vi "Saturation transfer-v2.vi"() -> ()   [LabVIEW 2016]
uses:
  <vilib>/Analysis/6fits.llb/Curve Fitting Criteria.ctl
  <vilib>/Utility/file.llb/Write To Spreadsheet File (string).vi
  <vilib>/Utility/file.llb/Write To Spreadsheet File (DBL).vi
  Driver/New driver/Agilent 415X Series.lvlib
  <vilib>/Analysis/NI_AALPro.lvlib
panel:
  out "power":dbl
  in  "short int. time":dbl(knob)=0.00064 scale=8e-05..0.00056
  in  "integration time":i32(slide) scale=0.0..2.0
  out "error out":errorcluster
  out "error":i32
  in  "parameter bounds":T1={"amp min"=-inf, "amp max"=inf, "power min"=-inf, "power max"=inf, "offset min"=0.0, "offset max"=0.0}
  in  "Dielectric thickness (nm)":dbl
  in  "Dielectric constant":dbl
  in  "Channel length (mm)":dbl
  in  "Channel width (mm)":dbl
  out "Graph  3":cluster{"Output data":dbl[], dbl[]}(graph) caption="Mobility Calculation"
  out "Graph  2":cluster{"Output data":dbl[], dbl[]}[](graph) caption="SMU 2 (ID) & SMU 3 (IG)"
  in  "LINEAR STEP":dbl
  in  "STOP":dbl
  in  "START":dbl
  in  "RATIO":dbl
  in  "OFFSET":dbl
  in  "FILE PATH":path
  out "SPA VISA resource name  End":refnum<visa-resource-name>
  in  "SPA VISA resource name Start":refnum<visa-resource-name>="GPIB0::14::INSTR"
  in  "error in (no error)":errorcluster
  # "SMU 3: Gate \nSMU3 = SMU2*RATIO\n             +OFFSET"
  # "SMU 1: Source"
  # "Common"
  # "SMU 2: Drain"
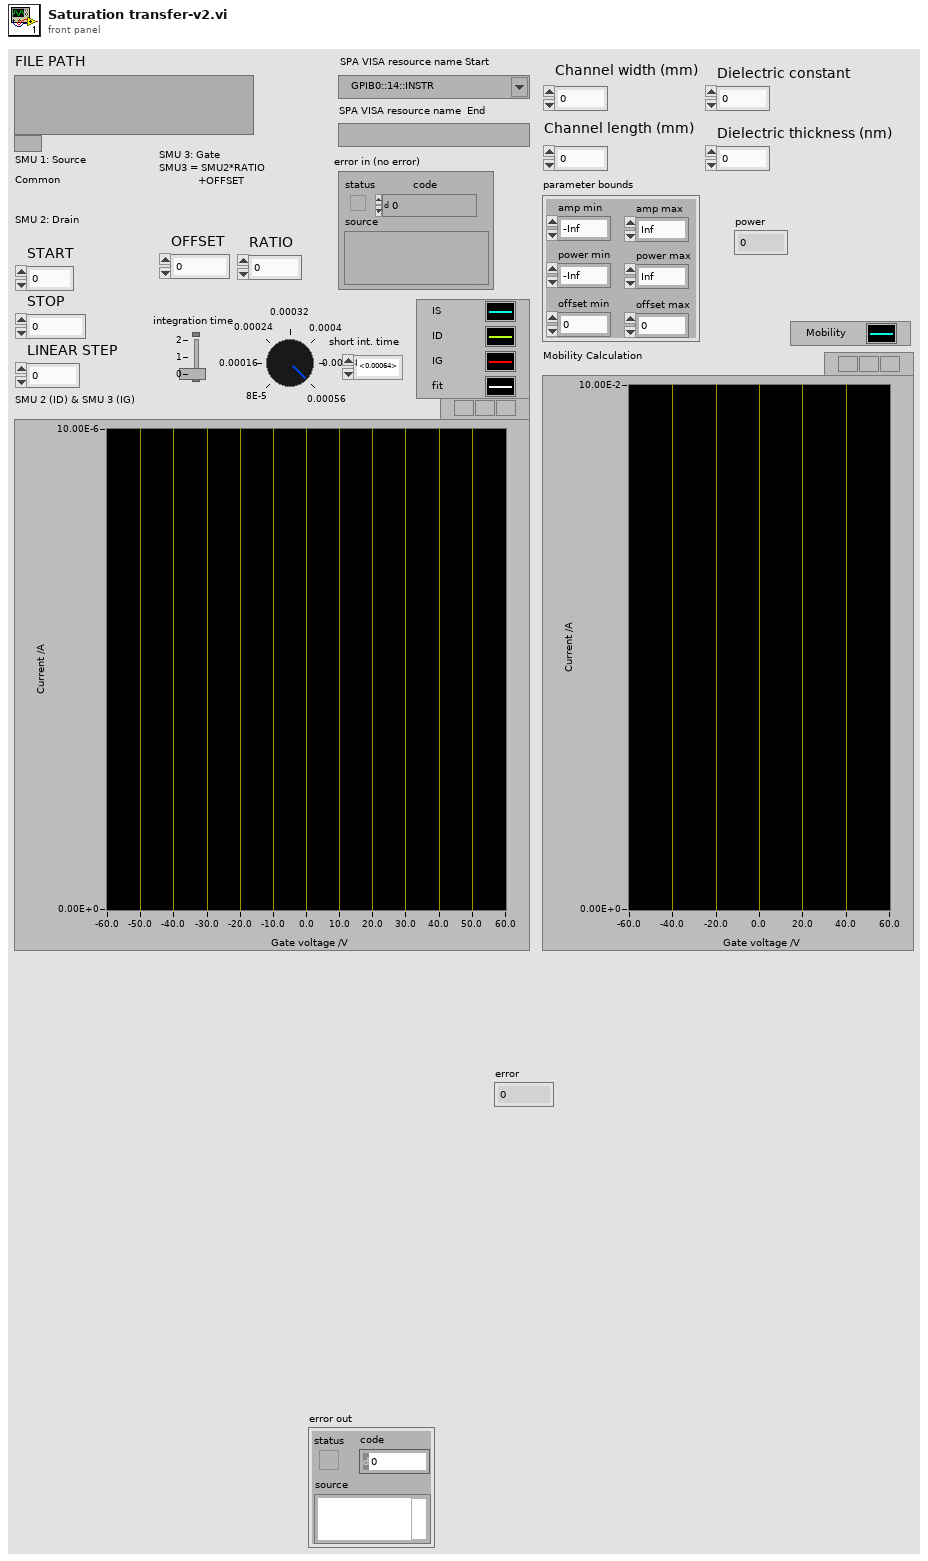
[diagram p1: front panel]
types:
  T1 = cluster{"amp min":dbl, "amp max":dbl, "power min":dbl, "power max":dbl, "offset min":dbl, "offset max":dbl}
  T2 = typedef "NI_AALPro.lvlib/Curve Fitting Criteria.ctl" = u16
  T3 = cluster{"Output data":dbl[], "Best Power Fit":dbl[]}[]
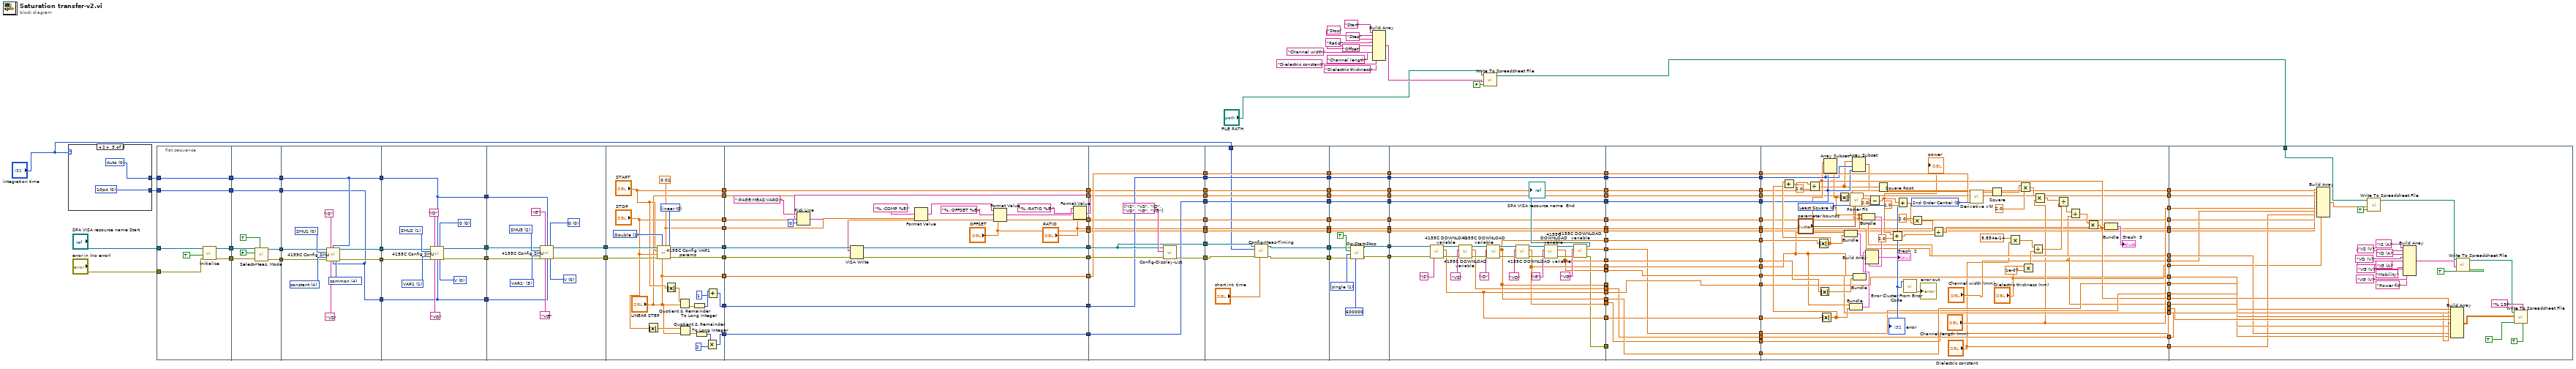
[diagram p0: block diagram]
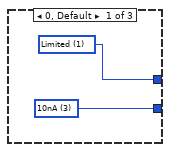
[diagram p2: hidden frame]
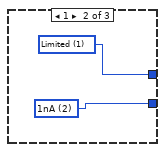
[diagram p3: hidden frame]
diagram:
  n1 = case shown="2" "integration time" {
    tunnel: [w143 w145 w147] -> w8
    tunnel: [w142 w144 w146] -> w4
    frame 0, Default {
      w142 = u8 3 items=["10pA  ", "100pA  ", "1nA  ", "10nA", "100nA", "1uA", "10uA", "100uA", "1mA", "10mA", "100mA", "1A"] ("Range")
      w143 = u16 1 items=["Auto", "Limited", "Fixed"] ("Range mode")
    }
    frame 1 {
      w144 = u8 2 items=["10pA  ", "100pA  ", "1nA  ", "10nA", "100nA", "1uA", "10uA", "100uA", "1mA", "10mA", "100mA", "1A"] ("Range")
      w145 = u16 1 items=["Auto", "Limited", "Fixed"] ("Range mode")
    }
    frame 2 {
      w146 = u8 0 items=["10pA  ", "100pA  ", "1nA  ", "10nA", "100nA", "1uA", "10uA", "100uA", "1mA", "10mA", "100mA", "1A"] ("Range")
      w147 = u16 0 items=["Auto", "Limited", "Fixed"] ("Range mode")
    }
  }
  n2 = flat-sequence {
    tunnel: "error in (no error)" -> [w153]
    tunnel: "SPA VISA resource name Start" -> [w152]
    tunnel: [w151] -> w141
    tunnel: [w150] -> w140
    tunnel: w8 -> [w149]
    tunnel: [w149] -> w7
    tunnel: w4 -> [w148]
    tunnel: [w148] -> w2
    tunnel: w141 -> [w162]
    tunnel: w140 -> [w161]
    tunnel: [w158] -> w139
    tunnel: [w157] -> w138
    tunnel: w7 -> [w156]
    tunnel: [w156] -> w6
    tunnel: [w155] -> w3
    tunnel: w2 -> [w155]
    tunnel: w139 -> [w168]
    tunnel: w138 -> [w166]
    tunnel: [w167] -> w133
    tunnel: [w165] -> w132
    tunnel: [w163] -> w114
    tunnel: w6 -> [w164]
    tunnel: [w164] -> w5
    tunnel: w3 -> [w163]
    tunnel: [w185] -> w137
    tunnel: [w184] -> w136
    tunnel: w133 -> [w178]
    tunnel: w132 -> [w177]
    tunnel: [w174] -> w118
    tunnel: w114 -> [w175]
    tunnel: [w175] -> w113
    tunnel: w5 -> [w174]
    tunnel: w136 -> [w191]
    tunnel: w137 -> [w192]
    tunnel: [w189] -> w131
    tunnel: [w188] -> w130
    tunnel: w118 -> [w187]
    tunnel: w113 -> [w186]
    tunnel: w131 -> [w217]
    tunnel: w130 -> [w216]
    tunnel: [w213] -> w117
    tunnel: [w212] -> w116
    tunnel: [w211] -> w115
    tunnel: ["LINEAR STEP"] -> w95
    tunnel: [w201] -> w88
    tunnel: [w206] -> w81
    tunnel: ["START"] -> w45
    tunnel: ["STOP"] -> w37
    tunnel: ["LINEAR STEP"] -> w29
    tunnel: w117 -> [w237]
    tunnel: [w236] -> w108
    tunnel: w116 -> [w239]
    tunnel: [w238] -> w107
    tunnel: w115 -> [w233]
    tunnel: [w225] -> w96
    tunnel: w95 -> [w225]
    tunnel: [w224] -> w89
    tunnel: w88 -> [w224]
    tunnel: [w223] -> w82
    tunnel: w81 -> [w223]
    tunnel: [w222] -> w46
    tunnel: w45 -> [w222]
    tunnel: [w221] -> w38
    tunnel: w37 -> [w221]
    tunnel: [w220] -> w30
    tunnel: w29 -> [w220]
    tunnel: ["RATIO"] -> w22
    tunnel: ["OFFSET"] -> w15
    tunnel: w108 -> [w248]
    tunnel: w107 -> [w249]
    tunnel: [w250] -> w106
    tunnel: [w248] -> w105
    tunnel: [w247] -> w97
    tunnel: w96 -> [w247]
    tunnel: [w246] -> w90
    tunnel: w89 -> [w246]
    tunnel: [w245] -> w83
    tunnel: w82 -> [w245]
    tunnel: [w244] -> w47
    tunnel: w46 -> [w244]
    tunnel: [w243] -> w39
    tunnel: w38 -> [w243]
    tunnel: [w242] -> w31
    tunnel: w30 -> [w242]
    tunnel: [w241] -> w23
    tunnel: w22 -> [w241]
    tunnel: [w240] -> w16
    tunnel: w15 -> [w240]
    tunnel: w106 -> [w255]
    tunnel: w105 -> [w257]
    tunnel: [w265] -> w98
    tunnel: w97 -> [w265]
    tunnel: [w264] -> w91
    tunnel: w90 -> [w264]
    tunnel: [w263] -> w84
    tunnel: w83 -> [w263]
    tunnel: [w262] -> w48
    tunnel: w47 -> [w262]
    tunnel: [w261] -> w40
    tunnel: w39 -> [w261]
    tunnel: [w260] -> w32
    tunnel: w31 -> [w260]
    tunnel: [w259] -> w24
    tunnel: w23 -> [w259]
    tunnel: [w258] -> w17
    tunnel: w16 -> [w258]
    tunnel: [w256] -> w10
    tunnel: [w254] -> w9
    tunnel: "integration time" -> [w253]
    tunnel: [w277] -> w110
    tunnel: [w276] -> w109
    tunnel: [w275] -> w99
    tunnel: w98 -> [w275]
    tunnel: [w274] -> w92
    tunnel: w91 -> [w274]
    tunnel: [w273] -> w85
    tunnel: w84 -> [w273]
    tunnel: [w272] -> w49
    tunnel: w48 -> [w272]
    tunnel: [w271] -> w41
    tunnel: w40 -> [w271]
    tunnel: [w270] -> w33
    tunnel: w32 -> [w270]
    tunnel: [w269] -> w25
    tunnel: w24 -> [w269]
    tunnel: [w268] -> w18
    tunnel: w17 -> [w268]
    tunnel: w10 -> [w267]
    tunnel: w9 -> [w266]
    tunnel: [w289] -> w129
    tunnel: [w296] -> w128
    tunnel: [w293] -> w127
    tunnel: [w295] -> w126
    tunnel: [w294] -> w125
    tunnel: [w298] -> w124
    tunnel: [w293] -> w123
    tunnel: [w295] -> w121
    tunnel: [w294] -> w119
    tunnel: [w293] -> w112
    tunnel: w110 -> [w292]
    tunnel: w109 -> [w291]
    tunnel: [w290] -> w104
    tunnel: [w289] -> w102
    tunnel: [w288] -> w100
    tunnel: w99 -> [w288]
    tunnel: [w287] -> w93
    tunnel: w92 -> [w287]
    tunnel: [w286] -> w86
    tunnel: w85 -> [w286]
    tunnel: [w285] -> w50
    tunnel: w49 -> [w285]
    tunnel: [w284] -> w42
    tunnel: w41 -> [w284]
    tunnel: [w283] -> w34
    tunnel: w33 -> [w283]
    tunnel: [w282] -> w26
    tunnel: w25 -> [w282]
    tunnel: [w281] -> w19
    tunnel: w18 -> [w281]
    tunnel: w129 -> [w325]
    tunnel: w128 -> [w324]
    tunnel: w127 -> [w323]
    tunnel: w126 -> [w322]
    tunnel: w125 -> [w321]
    tunnel: w124 -> [w320]
    tunnel: w123 -> [_]
    tunnel: [w332] -> w122
    tunnel: w121 -> [w332]
    tunnel: [w331] -> w120
    tunnel: w119 -> [w331]
    tunnel: w112 -> [w330]
    tunnel: [w330] -> w111
    tunnel: w104 -> [_]
    tunnel: [w329] -> w103
    tunnel: w102 -> [w329]
    tunnel: [w328] -> w101
    tunnel: w100 -> [w328]
    tunnel: [w327] -> w94
    tunnel: w93 -> [w327]
    tunnel: [w326] -> w87
    tunnel: w86 -> [w326]
    tunnel: [w325] -> w79
    tunnel: [w324] -> w77
    tunnel: [w323] -> w75
    tunnel: [w322] -> w73
    tunnel: [w321] -> w71
    tunnel: [w320] -> w69
    tunnel: [w319] -> w51
    tunnel: w50 -> [w319]
    tunnel: [w318] -> w43
    tunnel: w42 -> [w318]
    tunnel: [w317] -> w35
    tunnel: w34 -> [w317]
    tunnel: [w316] -> w27
    tunnel: w26 -> [w316]
    tunnel: [w315] -> w20
    tunnel: w19 -> [w315]
    tunnel: w122 -> [w345]
    tunnel: w120 -> [w398]
    tunnel: w111 -> [w399]
    tunnel: w103 -> [w395]
    tunnel: w101 -> [w383]
    tunnel: w94 -> [w359]
    tunnel: w87 -> [w358]
    tunnel: [w354] -> w80
    tunnel: w79 -> [w354]
    tunnel: [w353] -> w78
    tunnel: w77 -> [w353]
    tunnel: [w352] -> w76
    tunnel: w75 -> [w352]
    tunnel: [w351] -> w74
    tunnel: w73 -> [w351]
    tunnel: [w350] -> w72
    tunnel: w71 -> [w350]
    tunnel: [w349] -> w70
    tunnel: w69 -> [w349]
    tunnel: [w348] -> w68
    tunnel: [w347] -> w67
    tunnel: [w346] -> w66
    tunnel: [w344] -> w52
    tunnel: w51 -> [w344]
    tunnel: [w343] -> w44
    tunnel: w43 -> [w343]
    tunnel: [w342] -> w36
    tunnel: w35 -> [w342]
    tunnel: [w341] -> w28
    tunnel: w27 -> [w341]
    tunnel: [w340] -> w21
    tunnel: w20 -> [w340]
    tunnel: ["Channel width (mm)"] -> w14
    tunnel: ["Channel length (mm)"] -> w13
    tunnel: ["Dielectric constant"] -> w12
    tunnel: ["Dielectric thickness (nm)"] -> w11
    tunnel: w80 -> [w433]
    tunnel: w78 -> [w432]
    tunnel: w76 -> [w431]
    tunnel: w74 -> [w430]
    tunnel: w72 -> [w429]
    tunnel: w70 -> [w428]
    tunnel: w68 -> [w427]
    tunnel: w67 -> [w426]
    tunnel: w66 -> [w425]
    tunnel: w53 -> [w402]
    tunnel: w52 -> [w412]
    tunnel: w44 -> [w411]
    tunnel: w36 -> [w410]
    tunnel: w28 -> [w409]
    tunnel: w21 -> [w408]
    tunnel: w14 -> [w407]
    tunnel: w13 -> [w406]
    tunnel: w12 -> [w405]
    tunnel: w11 -> [w404]
    frame #0 {
      n3 = call "Initialize.vi"("error in (no error)"=w153, "reset"=TRUE, "VISA resource name"=w152) -> ("error out"=w150:errorcluster, "VISA resource name out"=w151:refnum<visa-resource-name>)  [unwired: 2 in, 5 out]
    }
    frame #1 {
      n4 = call "Select-Meas. Mode.vi"("clear all channels"=TRUE, "error in (no error)"=w161, "measurement mode"=FALSE, "VISA resource name"=w162) -> ("error out"=w157:errorcluster, "VISA resource name out"=w158:refnum<visa-resource-name>)  [unwired: 1 in, 5 out]
    }
    frame #2 {
      w169 = u32 0 items=["SMU1  ", "SMU2  ", "SMU3  ", "SMU4  ", "SMU5  ", "SMU6  "] ("unit to configure")
      w170 = u32 4 items=["disabled  ", "VAR1  ", "VAR2  ", "VAR1'  ", "constant  "] ("function")
      w171 = u32 4 items=["V  ", "I  ", "V pulse  ", "I pulse  ", "  common  "] ("mode")
      n5 = call "4155C Config SMU.vi"("VISA session"=w168, "I name (max 6 chars)"="IS", "Range mode"=w164, "unit to configure"=w169, "function"=w170, "error in (no error)"=w166, "V name (max 6 chars)"="VS", "Range"=w163, "mode"=w171) -> ("dup VISA resource name"=w167:refnum<visa-resource-name>, "error out"=w165:errorcluster)  [unwired: 5 in]
    }
    frame #3 {
      w176 = u32 0 items=["0  ", "10K Ohms  ", "100K Ohms  ", "1M Ohms  "] ("series resistance *")
      w179 = u32 1 items=["SMU1  ", "SMU2  ", "SMU3  ", "SMU4  ", "SMU5  ", "SMU6  "] ("unit to configure")
      w180 = u32 1 items=["disabled  ", "VAR1  ", "VAR2  ", "VAR1'  ", "constant  "] ("function")
      w181 = u32 0 items=["V  ", "I  ", "V pulse  ", "I pulse  ", "  common  "] ("mode")
      n6 = call "4155C Config SMU.vi"("VISA session"=w178, "I name (max 6 chars)"="ID", "Range mode"=w174, "series resistance *"=w176, "unit to configure"=w179, "function"=w180, "error in (no error)"=w177, "V name (max 6 chars)"="VD", "Range"=w175, "mode"=w181) -> ("dup VISA resource name"=w185:refnum<visa-resource-name>, "error out"=w184:errorcluster)  [unwired: 4 in]
    }
    frame #4 {
      w190 = u32 0 items=["0  ", "10K Ohms  ", "100K Ohms  ", "1M Ohms  "] ("series resistance *")
      w193 = u32 2 items=["SMU1  ", "SMU2  ", "SMU3  ", "SMU4  ", "SMU5  ", "SMU6  "] ("unit to configure")
      w194 = u32 3 items=["disabled  ", "VAR1  ", "VAR2  ", "VAR1'  ", "constant  "] ("function")
      w195 = u32 0 items=["V  ", "I  ", "V pulse  ", "I pulse  ", "  common  "] ("mode")
      n7 = call "4155C Config SMU.vi"("VISA session"=w192, "I name (max 6 chars)"="IG", "Range mode"=w187, "series resistance *"=w190, "unit to configure"=w193, "function"=w194, "error in (no error)"=w191, "V name (max 6 chars)"="VG", "Range"=w186, "mode"=w195) -> ("dup VISA resource name"=w189:refnum<visa-resource-name>, "error out"=w188:errorcluster)  [unwired: 4 in]
    }
    frame #5 {
      w211 = 0.01 ("compliance")
      w214 = u16 1 items=["Single", "Double"] ("sweep mode")
      w215 = u16 0 items=["linear", "log 10", "log 25", "log 50"] ("sweep spacing (linear: 0)")
      n8 = Absolute Value(x="STOP") -> (abs(x)=w204:dbl)
      n9 = call "4155C Config VAR1 params.vi"("sweep spacing (linear: 0)"=w215, "compliance"=w211, "step (linear only)"="LINEAR STEP", "sweep mode"=w214, "error in (no error)"=w216, "stop"="STOP", "start"="START", "VISA session"=w217) -> ("error out"=w212:errorcluster, "dup VISA resource name"=w213:refnum<visa-resource-name>)  [unwired: 1 in, 1 out]
      n10 = Absolute Value(x="START") -> (abs(x)=w205:dbl)
      n11 = Quotient & Remainder(x=w205, y="LINEAR STEP") -> (floor(x/y)=w210:dbl)  [unwired: 1 out]
      n12 = Quotient & Remainder(x=w204, y="LINEAR STEP") -> (floor(x/y)=w209:dbl)  [unwired: 1 out]
      n13 = To Long Integer(number=w210) -> (32bit integer=w203:i32)
      n14 = To Long Integer(number=w209) -> (32bit integer=w208:i32)
      n15 = Multiply(x=w208, y=2) -> (x*y=w206:i32)
      n16 = Add(x=w203, y=1) -> (x+y=w201:i32)
    }
    frame #6 {
      n17 = Format Value(format string="%.;COMP %E;", value (0)=w233) -> (output string=w227:string)  [unwired: 1 in]
      n18 = Format Value(string ("")=w227, format string="%.;OFFSET %E;", value (0)="OFFSET") -> (output string=w228:string)
      n19 = Format Value(string ("")=w228, format string="%.;RATIO %E;", value (0)="RATIO") -> (output string=w226:string)
      n20 = Pick Line(string ("")=":PAGE:MEAS:VARD:" ("write buffer (\"\")"), multi-line string=w226, line index=0) -> (output string=w232:string)
      n21 = VISA Write(VISA resource name=w237, write buffer=w232, error in (no error)=w239) -> (VISA resource name out=w236:refnum<visa-resource-name>, error out=w238:errorcluster)  [unwired: 1 out]
    }
    frame #7 {
      n22 = call "Config-Display-List.vi"("error in (no error)"=w249, "list (max 8 elements)"=string[] ["IS", "VS", "ID", "VD", "IG", "VG"], "VISA session"=w248) -> ("error out"=w250:errorcluster)  [unwired: 1 in, 7 out]
    }
    frame #8 {
      n23 = call "Config-Meas-Timing.vi"("short integration time\n(rounded to the nearest multiple of 80us)"="short int. time", "error in (no error)"=w255, "integration time"=w253, "VISA session"=w257) -> ("error out"=w254:errorcluster, "VISA resource name out"=w256:refnum<visa-resource-name>)  [unwired: 6 in]
    }
    frame #9 {
      w279 = 1 items=["stop  ", "single  ", "single-append  ", "stress start  ", "continuous  ", "standby on  ", "standby off  ", "zero  "] ("function (stop:0)")
      n24 = call "Op-Start-Stop.vi"("time to wait (30000ms)"=600000, "error in (no error)"=w266, "function (stop:0)"=w279, "wait until finish"=TRUE, "VISA resource name"=w267) -> ("error out"=w276:errorcluster, "VISA resource name out"=w277:refnum<visa-resource-name>)  [unwired: 5 out]
    }
    frame #10 {
      n25 = call "4155C DOWNLOAD variable.vi"("error in (no error)"=w291, "Variable name"="IS", "VISA resource name in"=w292) -> ("error out"=w314:errorcluster, "Output data"=w289:dbl[], "VISA Resource Name out"=w313:refnum<visa-resource-name>)  [unwired: 2 out]
      n26 = call "4155C DOWNLOAD variable.vi"("error in (no error)"=w314, "Variable name"="VS", "VISA resource name in"=w313) -> ("error out"=w311:errorcluster, "Output data"=w296:dbl[], "VISA Resource Name out"=w312:refnum<visa-resource-name>)  [unwired: 2 out]
      n27 = call "4155C DOWNLOAD variable.vi"("error in (no error)"=w311, "Variable name"="ID", "VISA resource name in"=w312) -> ("error out"=w303:errorcluster, "Output data"=w293:dbl[], "VISA Resource Name out"=w302:refnum<visa-resource-name>)  [unwired: 2 out]
      n28 = call "4155C DOWNLOAD variable.vi"("error in (no error)"=w303, "Variable name"="VD", "VISA resource name in"=w302) -> ("error out"=w306:errorcluster, "Output data"=w295:dbl[], "VISA Resource Name out"=w307:refnum<visa-resource-name>)  [unwired: 2 out]
      n29 = call "4155C DOWNLOAD variable.vi"("error in (no error)"=w306, "Variable name"="IG", "VISA resource name in"=w307) -> ("error out"=w300:errorcluster, "Output data"=w294:dbl[], "VISA Resource Name out"=w299:refnum<visa-resource-name>)  [unwired: 2 out]
      n30 = call "4155C DOWNLOAD variable.vi"("error in (no error)"=w300, "Variable name"="VG", "VISA resource name in"=w299) -> ("error out"=w290:errorcluster, "Output data"=w298:dbl[], "VISA Resource Name out"=→"SPA VISA resource name  End":refnum<visa-resource-name>)  [unwired: 2 out]
    }
    frame #11 {
    }
    frame #12 {
      w384 = u16 0 items=["2nd Order Central", "4th Order Central", "Forward", "Backward"] ("method")
      w387 = T2 0 items=["Least Square", "Least Absolute Residual", "Bisquare"] ("method")
      n31 = Absolute Value(x=w399) -> (abs(x)=w389:dbl[])
      n32 = Absolute Value(x=w398) -> (abs(x)=w397:dbl[])
      n33 = Absolute Value(x=w395) -> (abs(x)=w388:dbl[])
      n34 = Add(x=w389, y=w388) -> (x+y=w390:dbl[])
      n35 = Divide(x=w390, y=2.0) -> (x/y=w357:dbl[])
      n36 = Array Subset(array=w345, index=w359, length=w358) -> (w347:dbl[])
      n37 = Absolute Value(x=w347) -> (abs(x)=w355:dbl[])
      n38 = Bundle("Output data"=w345, w389) -> (w393:cluster{"Output data":dbl[], dbl[]})  [unwired: 1 in]
      n39 = Bundle("Output data"=w345, w388) -> (w394:cluster{"Output data":dbl[], dbl[]})  [unwired: 1 in]
      n40 = Array Subset(array=w357, index=w359, length=w358) -> (w356:dbl[])
      n41 = call <vilib>:"Power Fit.vi"("Y"=w356, "X"=w355, "method"=w387, "parameter bounds"="parameter bounds") -> ("Best Power Fit"=w346:dbl[], "power"=w335:dbl, "error"=w361:i32)  [unwired: 6 in, 3 out]
      "error" <- w361
      n42 = Bundle("Output data"=w345, w397) -> (w392:cluster{"Output data":dbl[], dbl[]})  [unwired: 1 in]
      n43 = Bundle(w347, "Best Power Fit"=w346) -> (w386:cluster{dbl[], "Best Power Fit":dbl[]})  [unwired: 1 in]
      n44 = Build Array(w394, w393, w392, w386) -> (→"Graph  2":T3)
      n45 = Subtract(x=w335, y=2.0) -> (x-y=w333:dbl)
      "power" <- w333
      n46 = Square Root(x=w357) -> (sqrt(x)=w382:dbl[])
      n47 = Add(x=w333, y=2.0) -> (x+y=w364:dbl)
      n48 = Add(x=w333, y=1.0) -> (x+y=w366:dbl)
      n49 = call <vilib>:"Error Cluster From Error Code.vi"("error code (0)"=w361) -> ("error out"=→"error out":errorcluster)  [unwired: 8 in]
      n50 = Multiply(x=2.0, y=w366) -> (x*y=w365:dbl)
      n51 = Divide(x=w365, y=w364) -> (x/y=w363:dbl)
      n52 = call <vilib>:"Derivative x(t).vi"("method"=w384, "dt"=w383, "X"=w382) -> ("dX/dt"=w381:dbl[])  [unwired: 7 in, 1 out]
      n53 = Square(x=w381) -> (x^2=w376:dbl[])
      n54 = Multiply(x=8.854e-14, y="Dielectric constant") -> (x*y=w379:dbl)
      n55 = Multiply(x=w376, y=2.0) -> (x*y=w374:dbl[])
      n56 = Multiply(x="Dielectric thickness (nm)", y=1e-07) -> (x*y=w377:dbl)
      n57 = Divide(x=w379, y=w377) -> (x/y=w373:dbl)
      n58 = Multiply(x=w374, y="Channel length (mm)") -> (x*y=w372:dbl[])
      n59 = Divide(x=w372, y=w373) -> (x/y=w371:dbl[])
      n60 = Divide(x=w371, y="Channel width (mm)") -> (x/y=w370:dbl[])
      n61 = Multiply(x=w370, y=w363) -> (x*y=w348:dbl[])
      n62 = Bundle("Output data"=w345, w348) -> (→"Graph  3":cluster{"Output data":dbl[], dbl[]})  [unwired: 1 in]
    }
    frame #13 {
      n63 = Build Array(w412, w411, w410, w409, w408, w407, w406, w405, w404) -> (w403:dbl[])
      n64 = call-poly <vilib>:"Write To Spreadsheet File.vi"("append to file? (new file:F)"=TRUE, "1D data"=w403, "file path (dialog if empty)"=w402) -> ("new file path (Not A Path if cancelled)"=w400:path)  [unwired: 5 in]
      n65 = Build Array("IS (A)" ("string"), "VS (V)" ("string"), "ID (A)" ("string"), "VD (V)" ("string"), "IG (A)" ("string"), "VG (V)" ("string"), "Mobility" ("element"), "VG (V)" ("element"), "Power fit" ("element")) -> (w414:string[])
      n66 = Build Array(w433, w432, w431, w430, w429, w428, w427, w426, w425) -> (w434:dbl[][])
      n67 = call-poly <vilib>:"Write To Spreadsheet File.vi"("append to file? (new file:F)"=TRUE, "1D data"=w414, "file path (dialog if empty)"=w400) -> ("new file path (Not A Path if cancelled)"=w413:path)  [unwired: 5 in]
      n68 = call-poly <vilib>:"Write To Spreadsheet File.vi"("transpose? (no:F)"=TRUE, "format (%.3f)"="%.13f", "append to file? (new file:F)"=TRUE, "2D data"=w434, "file path (dialog if empty)"=w413) -> ()  [unwired: 1 in, 3 out]
    }
  }
  n69 = Build Array("Start" ("string"), "Stop" ("string"), "Step" ("string"), "Ratio" ("string"), "Offset" ("string"), "Channel width" ("string"), "Channel length" ("element"), "Dielectric constant" ("element"), "Dielectric thickness" ("element")) -> (w58:string[])
  n70 = call-poly <vilib>:"Write To Spreadsheet File.vi"("append to file? (new file:F)"=FALSE, "1D data"=w58, "file path (dialog if empty)"="FILE PATH") -> ("new file path (Not A Path if cancelled)"=w53:path)  [unwired: 5 in]
